vi "readMultiTherm.vi"(8 "error in":errorcluster, 9 "ThermalConfigs":T1[](array[typedef]) {"Last Temp Readings"."Ambient Temp (°F)" format="%.2f °F"; "Last Temp Readings"."Ambient Temp (°C)" format="%.2f °C"; "Last Temp Readings"."Object Temp (°F)" format="%.2f °F"; "Last Temp Readings"."Object Temp (°C)" format="%.2f °C"; "Samples to Average" items=["1 sample, .26s conversion"=0, "2 samples, .51s conversion"=512, "4 samples, 1.01s conversion"=1024, "8 samples, 2.01s conversion"=1536, "16 samples, 4.01s conversion"=2048]; "I2C Slave Address" format="%.0x"}, 11 "LINX Resource in":T3) -> (0 "error out":errorcluster, 1 "ThermalConfigs":T1[](array[typedef]) {"Last Temp Readings"."Ambient Temp (°F)" format="%.2f °F"; "Last Temp Readings"."Ambient Temp (°C)" format="%.2f °C"; "Last Temp Readings"."Object Temp (°F)" format="%.2f °F"; "Last Temp Readings"."Object Temp (°C)" format="%.2f °C"; "Samples to Average" items=["1 sample, .26s conversion"=0, "2 samples, .51s conversion"=512, "4 samples, 1.01s conversion"=1024, "8 samples, 2.01s conversion"=1536, "16 samples, 4.01s conversion"=2048]; "I2C Slave Address" format="%.0x"}, 2 "ThermReadings":T2[](array[typedef]) {"Ambient Temp (°F)" format="%.2f °F"; "Ambient Temp (°C)" format="%.2f °C"; "Object Temp (°F)" format="%.2f °F"; "Object Temp (°C)" format="%.2f °C"}, 3 "LINX Resource out":T3)   [LabVIEW 2017]
uses:
  Type Defs/thermopileSettings.ctl
  Type Defs/tempReadings.ctl
  <vilib>/MakerHub/LINX/Private/Type Defs/LINX Ref.ctl
  <vilib>/MakerHub/LINX/Private/Type Defs/Platform.ctl
  <vilib>/MakerHub/LINX/Private/Type Defs/Interface.ctl
  <vilib>/MakerHub/LINX/Private/Device/Type Defs/LINX Device Config.ctl
  <vilib>/MakerHub/LINX/Private/Device/Type Defs/TCP Config.ctl
  <vilib>/MakerHub/LINX/Private/Device/Type Defs/Channels.ctl
  <vilib>/MakerHub/LINX/LMH-LINX.lvlib
  <vilib>/MakerHub/LINX/Private/Device/Device.lvlib
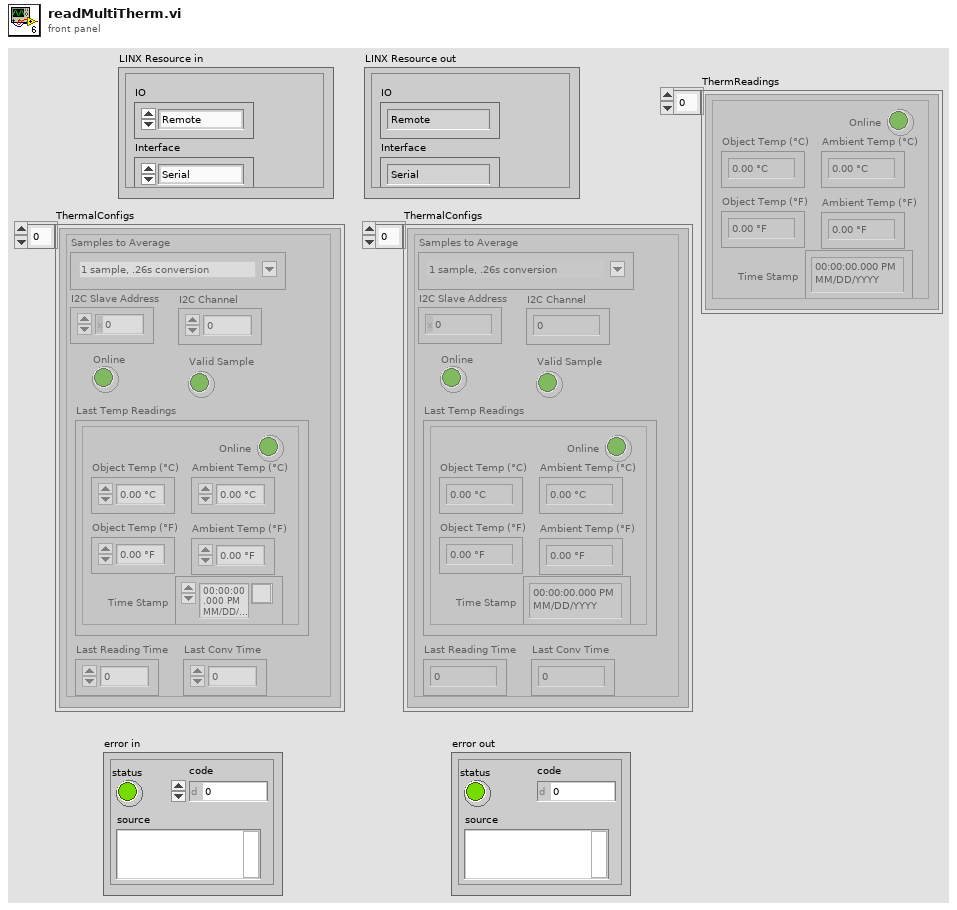
[diagram p1: front panel]
types:
  T1 = typedef "thermopileSettings.ctl" = cluster{"Online":bool, "I2C Channel":u8, "I2C Slave Address":u8, "Valid Sample":bool, "Samples to Average":u16, "Last Temp Readings":T2, "Last Reading Time":dbl, "Last Conv Time":dbl}
  T2 = typedef "tempReadings.ctl" = cluster{"Object Temp (°C)":dbl, "Object Temp (°F)":dbl, "Ambient Temp (°C)":dbl, "Ambient Temp (°F)":dbl, "Online":bool, "Time Stamp":timestamp}
  T3 = typedef "LMH-LINX.lvlib/LINX Ref.ctl" = cluster{"IO":T4, "Interface":T5, "LINX Device Config":T6}
  T4 = typedef "LMH-LINX.lvlib/Platform.ctl" = enum16{"Remote", "Local"}
  T5 = typedef "LMH-LINX.lvlib/Interface.ctl" = enum16{"Serial", "TCP"}
  T6 = typedef "LMH-LINX.lvlib/Device.lvlib/LINX Device Config.ctl" = cluster{"Interface":T5, "COM Port":refnum<visa-resource-name>, "TCP Configuration":T7, "Device Family":u8, "Device ID":u8, "Device Name":string, "TCP Ref":refnum<k5>, "Channels":T8}
  T7 = typedef "LMH-LINX.lvlib/Device.lvlib/TCP Config.ctl" = cluster{"IP Address":string, "Port":u16}
  T8 = typedef "LMH-LINX.lvlib/Channels.ctl" = cluster{"DI":u8[], "DO":u8[], "AI":u8[], "AO":u8[], "PWM":u8[], "QE":u8[], "UART":u8[], "I2C 2":u8[], "SPI":u8[], "CAN":u8[], "Servo":u8[], "AI Ref (V)":dbl, "AI Resolution (Bits)":u8, "AO Ref (V)":dbl, "AO Resolution (Bits)":u8}
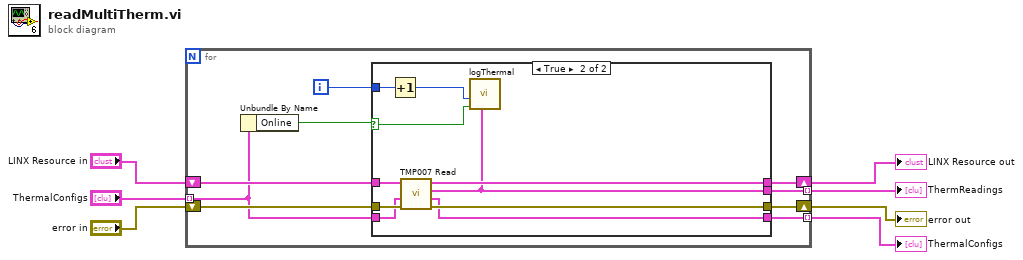
[diagram p0: block diagram]
diagram:
  n1 = for {
    tunnel: "ThermalConfigs" -> [w10] mode=indexing
    shift-right: [w13] -> w6
    shift-left: "LINX Resource in" -> [w16]
    shift-right: [w14] -> w5
    shift-left: "error in" -> [w15]
    tunnel: [w12] -> w4 mode=indexing
    tunnel: [w9] -> w7 mode=indexing
    i -> [w8]
    n2 = Unbundle By Name(w10) -> ("Online"=w11:bool)
    n3 = case shown="True" w11 {
      selector: w11 -> [_ w25]
      tunnel: w16 -> [w19 w29]
      tunnel: w15 -> [w18 w28]
      tunnel: [w18 w21] -> w14
      tunnel: [w19 w27] -> w13
      tunnel: [_ w24] -> w12
      tunnel: w10 -> [w17 w22]
      tunnel: [w17 w20] -> w9
      tunnel: w8 -> [_ w26]
      frame False {
      }
      frame True {
        n4 = Increment(x=w26) -> (x+1=w23:i32)
        n5 = call "TMP007 Read.vi"("error in (no error)"=w28, "Thermopile Setting"=w22, "LINX Resource in"=w29) -> ("error out"=w21:errorcluster, "Thermopile Status"=w20:T1, "Temp Readings"=w24:T2, "LINX Resource"=w27:T3)  [unwired: 4 in, 1 out]
        n6 = call "logThermal.vi"("Temp Readings"=w24, "Online"=w25, "Index"=w23) -> ()  [unwired: 9 in]
      }
    }
  }
  "ThermalConfigs" <- w7
  "LINX Resource out" <- w6
  "error out" <- w5
  "ThermReadings" <- w4
